vi "Initiate Stop.vi"(6 "error in (no error)":errorcluster, 8 "Loops":T1, 9 "Message Queues in":T2) -> (0 "error out":errorcluster)   [LabVIEW 2014]
uses:
  support/Message Queue/All Message Queues.ctl
  support/Message Queue/Message Cluster.ctl
  Loops.ctl
  support/Message Queue/Enqueue Message (Single).vi
  support/Message Queue/Message Queue.lvlib
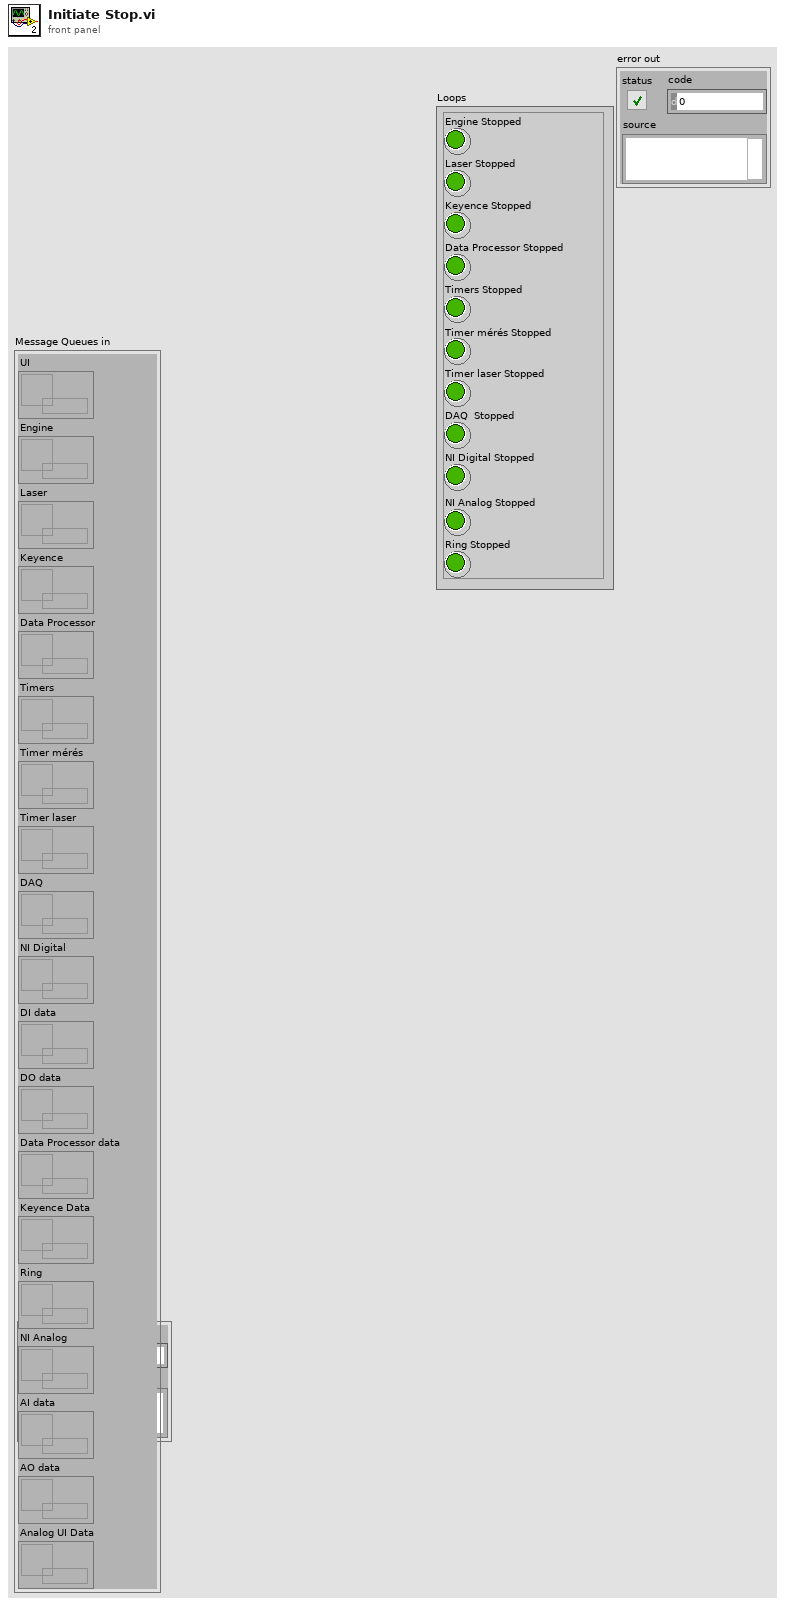
[diagram p1: front panel]
types:
  T1 = typedef "Loops.ctl" = cluster{"Engine Stopped":bool, "Laser Stopped":bool, "Keyence Stopped":bool, "Data Processor Stopped":bool, "Timers Stopped":bool, "Timer mérés Stopped":bool, "Timer laser Stopped":bool, "DAQ  Stopped":bool, "NI Digital Stopped":bool, "NI Analog Stopped":bool, "Ring Stopped":bool}
  T2 = typedef "Message Queue.lvlib/All Message Queues.ctl" = cluster{"UI":refnum<queue>, "Engine":refnum<queue>, "Laser":refnum<queue>, "Keyence":refnum<queue>, "Data Processor":refnum<queue>, "Timers":refnum<queue>, "Timer mérés":refnum<queue>, "Timer laser":refnum<queue>, "DAQ":refnum<queue>, "NI Digital":refnum<queue>, "DI data":refnum<queue>, "DO data":refnum<queue>, "Data Processor data":refnum<queue>, "Keyence Data":refnum<queue>, "Ring":refnum<queue>, "NI Analog":refnum<queue>, "AI data":refnum<queue>, "AO data":refnum<queue>, "Analog UI Data":refnum<queue>}
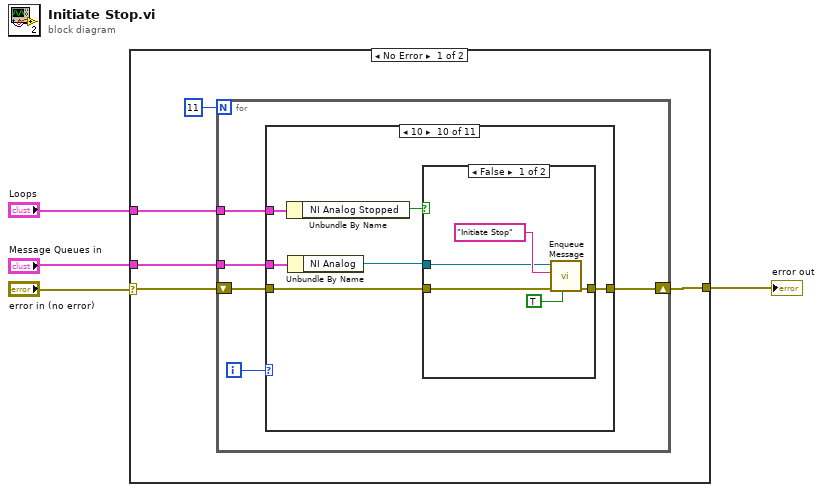
[diagram p0: block diagram]
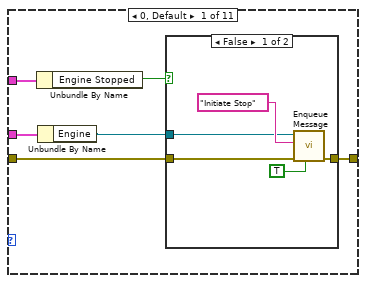
[diagram p2: hidden frame]
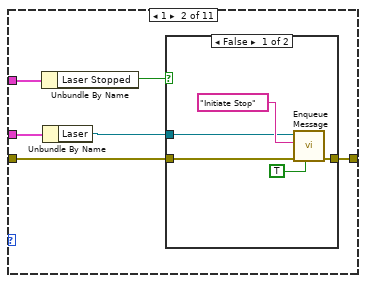
[diagram p4: hidden frame]
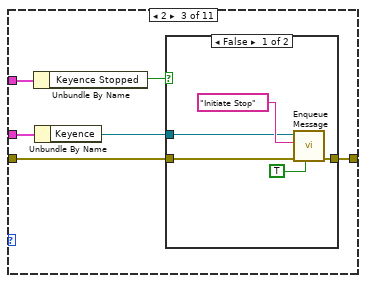
[diagram p6: hidden frame]
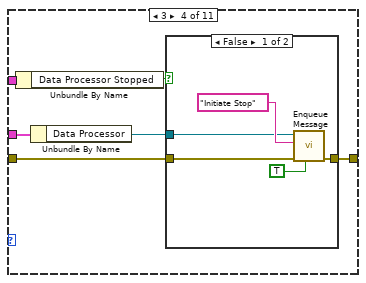
[diagram p8: hidden frame]
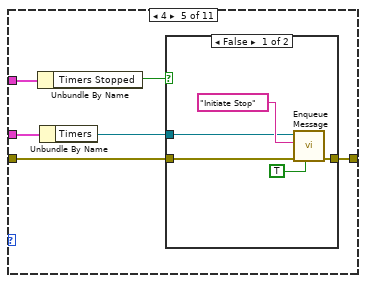
[diagram p10: hidden frame]
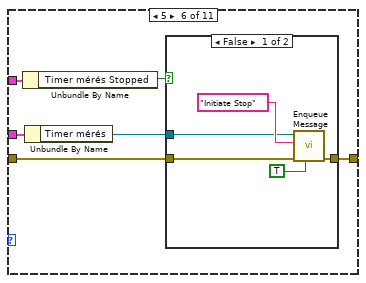
[diagram p12: hidden frame]
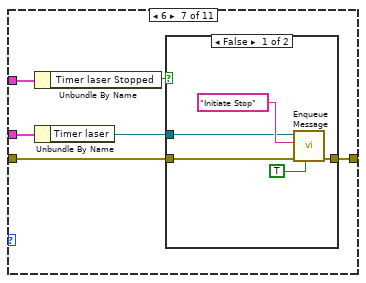
[diagram p14: hidden frame]
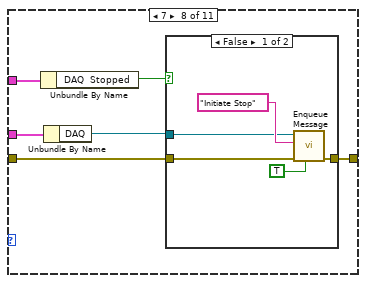
[diagram p16: hidden frame]
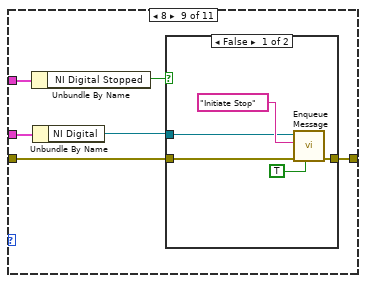
[diagram p18: hidden frame]
diagram:
  n1 = case shown="No Error" "error in (no error)" {
    selector: "error in (no error)" -> [w9 w147]
    tunnel: "Message Queues in" -> [w5 _]
    tunnel: [w7 w147] -> w1
    tunnel: "Loops" -> [w6 _]
    frame No Error {
      n2 = for {
        N: 11 -> [_]
        shift-right: [w14] -> w7
        shift-left: w9 -> [w13]
        tunnel: w6 -> [w11]
        tunnel: w5 -> [w10]
        i -> [w12]
        n3 = case shown="10" w12 {
          tunnel: w13 -> [w16 w28 w40 w52 w64 w76 w88 w100 w112 w124 w136]
          tunnel: w10 -> [w19 w31 w43 w55 w67 w79 w91 w103 w115 w127 w139]
          tunnel: [w15 w27 w39 w51 w63 w75 w87 w99 w111 w123 w135] -> w14
          tunnel: w11 -> [w20 w32 w44 w56 w68 w80 w92 w104 w116 w128 w140]
          frame 0, Default {
            n4 = Unbundle By Name(w20) -> ("Engine Stopped"=w17:bool)
            n5 = Unbundle By Name(w19) -> ("Engine"=w18:refnum<queue>)
            n6 = case shown="False" w17 {
              tunnel: w18 -> [w23 _]
              tunnel: w16 -> [w22 w26]
              tunnel: [w21 w26] -> w15
              frame False {
                n7 = call-poly "Enqueue Message.vi"("Priority Message? (F)"=TRUE, "error in (no error)"=w22, "Message"="Initiate Stop", "Message Queue"=w23) -> ("error out"=w21:errorcluster)  [unwired: 6 in, 1 out]
              }
              frame True {
              }
            }
          }
          frame 1 {
            n8 = Unbundle By Name(w32) -> ("Laser Stopped"=w29:bool)
            n9 = Unbundle By Name(w31) -> ("Laser"=w30:refnum<queue>)
            n10 = case shown="False" w29 {
              tunnel: w30 -> [w35 _]
              tunnel: w28 -> [w34 w38]
              tunnel: [w33 w38] -> w27
              frame False {
                n11 = call-poly "Enqueue Message.vi"("Priority Message? (F)"=TRUE, "error in (no error)"=w34, "Message"="Initiate Stop", "Message Queue"=w35) -> ("error out"=w33:errorcluster)  [unwired: 6 in, 1 out]
              }
              frame True {
              }
            }
          }
          frame 2 {
            n12 = Unbundle By Name(w44) -> ("Keyence Stopped"=w41:bool)
            n13 = Unbundle By Name(w43) -> ("Keyence"=w42:refnum<queue>)
            n14 = case shown="False" w41 {
              tunnel: w42 -> [w47 _]
              tunnel: w40 -> [w46 w50]
              tunnel: [w45 w50] -> w39
              frame False {
                n15 = call-poly "Enqueue Message.vi"("Priority Message? (F)"=TRUE, "error in (no error)"=w46, "Message"="Initiate Stop", "Message Queue"=w47) -> ("error out"=w45:errorcluster)  [unwired: 6 in, 1 out]
              }
              frame True {
              }
            }
          }
          frame 3 {
            n16 = Unbundle By Name(w56) -> ("Data Processor Stopped"=w53:bool)
            n17 = Unbundle By Name(w55) -> ("Data Processor"=w54:refnum<queue>)
            n18 = case shown="False" w53 {
              tunnel: w54 -> [w59 _]
              tunnel: w52 -> [w58 w62]
              tunnel: [w57 w62] -> w51
              frame False {
                n19 = call-poly "Enqueue Message.vi"("Priority Message? (F)"=TRUE, "error in (no error)"=w58, "Message"="Initiate Stop", "Message Queue"=w59) -> ("error out"=w57:errorcluster)  [unwired: 6 in, 1 out]
              }
              frame True {
              }
            }
          }
          frame 4 {
            n20 = Unbundle By Name(w68) -> ("Timers Stopped"=w65:bool)
            n21 = Unbundle By Name(w67) -> ("Timers"=w66:refnum<queue>)
            n22 = case shown="False" w65 {
              tunnel: w66 -> [w71 _]
              tunnel: w64 -> [w70 w74]
              tunnel: [w69 w74] -> w63
              frame False {
                n23 = call-poly "Enqueue Message.vi"("Priority Message? (F)"=TRUE, "error in (no error)"=w70, "Message"="Initiate Stop", "Message Queue"=w71) -> ("error out"=w69:errorcluster)  [unwired: 6 in, 1 out]
              }
              frame True {
              }
            }
          }
          frame 5 {
            n24 = Unbundle By Name(w80) -> ("Timer mérés Stopped"=w77:bool)
            n25 = Unbundle By Name(w79) -> ("Timer mérés"=w78:refnum<queue>)
            n26 = case shown="False" w77 {
              tunnel: w78 -> [w83 _]
              tunnel: w76 -> [w82 w86]
              tunnel: [w81 w86] -> w75
              frame False {
                n27 = call-poly "Enqueue Message.vi"("Priority Message? (F)"=TRUE, "error in (no error)"=w82, "Message"="Initiate Stop", "Message Queue"=w83) -> ("error out"=w81:errorcluster)  [unwired: 6 in, 1 out]
              }
              frame True {
              }
            }
          }
          frame 6 {
            n28 = Unbundle By Name(w92) -> ("Timer laser Stopped"=w89:bool)
            n29 = Unbundle By Name(w91) -> ("Timer laser"=w90:refnum<queue>)
            n30 = case shown="False" w89 {
              tunnel: w90 -> [w95 _]
              tunnel: w88 -> [w94 w98]
              tunnel: [w93 w98] -> w87
              frame False {
                n31 = call-poly "Enqueue Message.vi"("Priority Message? (F)"=TRUE, "error in (no error)"=w94, "Message"="Initiate Stop", "Message Queue"=w95) -> ("error out"=w93:errorcluster)  [unwired: 6 in, 1 out]
              }
              frame True {
              }
            }
          }
          frame 7 {
            n32 = Unbundle By Name(w104) -> ("DAQ  Stopped"=w101:bool)
            n33 = Unbundle By Name(w103) -> ("DAQ"=w102:refnum<queue>)
            n34 = case shown="False" w101 {
              tunnel: w102 -> [w107 _]
              tunnel: w100 -> [w106 w110]
              tunnel: [w105 w110] -> w99
              frame False {
                n35 = call-poly "Enqueue Message.vi"("Priority Message? (F)"=TRUE, "error in (no error)"=w106, "Message"="Initiate Stop", "Message Queue"=w107) -> ("error out"=w105:errorcluster)  [unwired: 6 in, 1 out]
              }
              frame True {
              }
            }
          }
          frame 8 {
            n36 = Unbundle By Name(w116) -> ("NI Digital Stopped"=w113:bool)
            n37 = Unbundle By Name(w115) -> ("NI Digital"=w114:refnum<queue>)
            n38 = case shown="False" w113 {
              tunnel: w114 -> [w119 _]
              tunnel: w112 -> [w118 w122]
              tunnel: [w117 w122] -> w111
              frame False {
                n39 = call-poly "Enqueue Message.vi"("Priority Message? (F)"=TRUE, "error in (no error)"=w118, "Message"="Initiate Stop", "Message Queue"=w119) -> ("error out"=w117:errorcluster)  [unwired: 6 in, 1 out]
              }
              frame True {
              }
            }
          }
          frame 10 {
            n40 = Unbundle By Name(w128) -> ("NI Analog Stopped"=w125:bool)
            n41 = Unbundle By Name(w127) -> ("NI Analog"=w126:refnum<queue>)
            n42 = case shown="False" w125 {
              tunnel: w126 -> [w131 _]
              tunnel: w124 -> [w130 w134]
              tunnel: [w129 w134] -> w123
              frame False {
                n43 = call-poly "Enqueue Message.vi"("Priority Message? (F)"=TRUE, "error in (no error)"=w130, "Message"="Initiate Stop", "Message Queue"=w131) -> ("error out"=w129:errorcluster)  [unwired: 6 in, 1 out]
              }
              frame True {
              }
            }
          }
          frame 9 {
            n44 = Unbundle By Name(w140) -> ("Ring Stopped"=w137:bool)
            n45 = Unbundle By Name(w139) -> ("Ring"=w138:refnum<queue>)
            n46 = case shown="False" w137 {
              tunnel: w138 -> [w143 _]
              tunnel: w136 -> [w142 w146]
              tunnel: [w141 w146] -> w135
              frame False {
                n47 = call-poly "Enqueue Message.vi"("Priority Message? (F)"=TRUE, "error in (no error)"=w142, "Message"="Initiate Stop", "Message Queue"=w143) -> ("error out"=w141:errorcluster)  [unwired: 6 in, 1 out]
              }
              frame True {
              }
            }
          }
        }
      }
    }
    frame Error {
    }
  }
  "error out" <- w1
